vi "Write Log File.vi"(8 "error in (no error)":errorcluster, 10 "Log File":path, 11 "Mag Lab Error Handler in":refnum<class "Mag Lab Error Handler.lvclass">) -> (0 "error out":errorcluster, 3 "Mag Lab Error Handler out":refnum<class "Mag Lab Error Handler.lvclass">)   [LabVIEW 2015, in "Mag Lab Error Handler.lvlib" / "Mag Lab Error Handler.lvclass"]
uses:
  Mag Lab Error Handler.lvclass
  Mag Lab Error Handler.lvclass/Mag Lab Error Handler.ctl
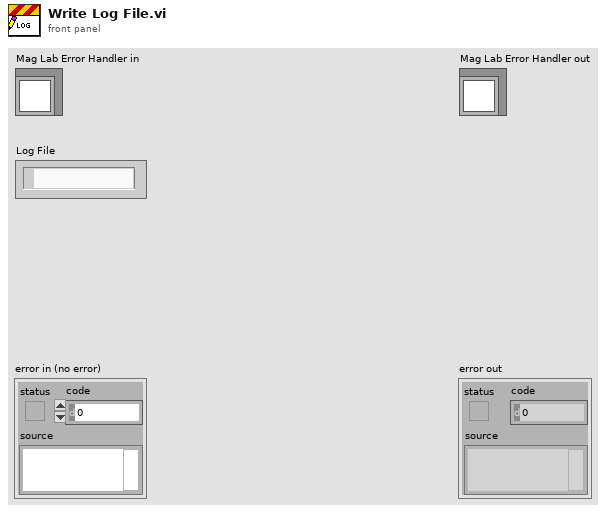
[diagram p1: front panel]
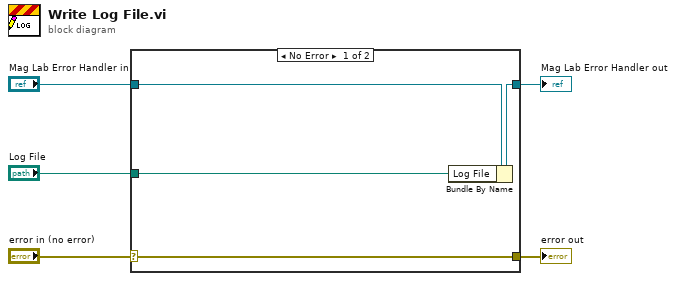
[diagram p0: block diagram]
diagram:
  n1 = case shown="No Error" "error in (no error)" {
    selector: "error in (no error)" -> [w9 w10]
    tunnel: [w9 w10] -> w4
    tunnel: [w7 w11] -> w2
    tunnel: "Mag Lab Error Handler in" -> [w8 w11]
    tunnel: "Log File" -> [w6 _]
    frame No Error {
      n2 = Bundle By Name(cluster=w8, "Log File"=w6) -> (w7:refnum<class "Mag Lab Error Handler.lvclass">)
    }
    frame Error {
    }
  }
  "error out" <- w4
  "Mag Lab Error Handler out" <- w2
